vi "7495_Fast.vi"(4 "Clk 1\nR-Shift":bool, 5 "Serial\nInput":bool, 6 "Clk 2\nL-Shift":bool, 7 "Mode\nControl":bool, 8 "D":bool, 9 "C":bool, 10 "B":bool, 11 "A":bool) -> (0 "OD":bool, 1 "OC":bool, 2 "OB":bool, 3 "OA":bool)   [LabVIEW 2012]
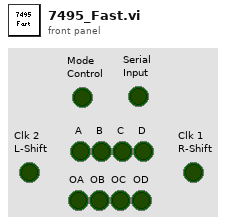
[diagram p1: front panel]
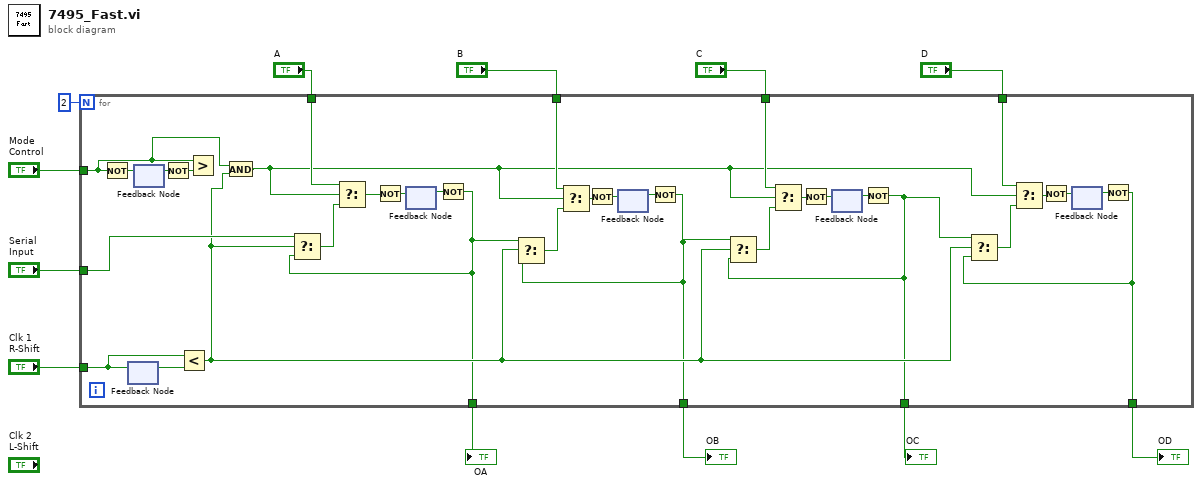
[diagram p0: block diagram]
diagram:
  n1 = for {
    N: 2 -> [_]
    tunnel: "A" -> [w45]
    tunnel: "B" -> [w43]
    tunnel: "C" -> [w41]
    tunnel: "D" -> [w39]
    tunnel: "Clk 1\nR-Shift" -> [w36]
    tunnel: "Serial\nInput" -> [w24]
    tunnel: "Mode\nControl" -> [w21]
    tunnel: [w19] -> w5
    tunnel: [w18] -> w4
    tunnel: [w15] -> w3
    tunnel: [w13] -> w2
    n2 = Not(x=w21) -> (.not. x?=w27:bool)
    n3 = feedback #1() -> (w37:bool)  [unwired: 1 in]
    n4 = feedback-in #1(w36) -> ()
    n5 = feedback #2() -> (w26:bool)  [unwired: 1 in]
    n6 = feedback-in #2(w27) -> ()
    n7 = Not(x=w26) -> (.not. x?=w25:bool)
    n8 = Less?(x=w36, y=w37) -> (x < y?=w23:bool)
    n9 = Greater?(x=w21, y=w25) -> ()  [unwired: 1 out]
    n10 = And(x=w21, y=w23) -> (x .and. y?=w22:bool)
    n11 = feedback #3() -> (w34:bool)  [unwired: 1 in]
    n12 = Not(x=w34) -> (.not. x?=w19:bool)
    n13 = Select(t=w24, s=w23, f=w19) -> (s? t:f=w38:bool)
    n14 = Select(t=w45, s=w22, f=w38) -> (s? t:f=w20:bool)
    n15 = Not(x=w20) -> (.not. x?=w35:bool)
    n16 = feedback-in #3(w35) -> ()
    n17 = feedback #4() -> (w33:bool)  [unwired: 1 in]
    n18 = Not(x=w33) -> (.not. x?=w18:bool)
    n19 = Select(t=w19, s=w23, f=w18) -> (s? t:f=w44:bool)
    n20 = Select(t=w43, s=w22, f=w44) -> (s? t:f=w17:bool)
    n21 = Not(x=w17) -> (.not. x?=w32:bool)
    n22 = feedback-in #4(w32) -> ()
    n23 = feedback #5() -> (w30:bool)  [unwired: 1 in]
    n24 = Not(x=w30) -> (.not. x?=w15:bool)
    n25 = Select(t=w18, s=w23, f=w15) -> (s? t:f=w42:bool)
    n26 = Select(t=w41, s=w22, f=w42) -> (s? t:f=w16:bool)
    n27 = Not(x=w16) -> (.not. x?=w31:bool)
    n28 = feedback-in #5(w31) -> ()
    n29 = feedback #6() -> (w29:bool)  [unwired: 1 in]
    n30 = Not(x=w29) -> (.not. x?=w13:bool)
    n31 = Select(t=w15, s=w23, f=w13) -> (s? t:f=w40:bool)
    n32 = Select(t=w39, s=w22, f=w40) -> (s? t:f=w14:bool)
    n33 = Not(x=w14) -> (.not. x?=w28:bool)
    n34 = feedback-in #6(w28) -> ()
  }
  "OA" <- w5
  "OB" <- w4
  "OC" <- w3
  "OD" <- w2
